vi "GetMoreGitInfoFromHash.vi"(10 "git hash":string, 11 "git hash file path":path=path "C:/Users/jmckenna/MIDAS_GEM_LabVIEW/.git/HEAD/refs/heads/master\n") -> (3 "git commit":T1, 4 "Full git text (before split into cluster)":string)   [LabVIEW 2018]
uses:
  GitCommitData.ctl
  <userlib>/_RADE/MTA-lib/file/file.llb/Valid Path - Traditional__ogtk.vi
  <userlib>/_RADE/MTA-lib/file/file.llb/Strip Path - Traditional__ogtk.vi
panel:
  out "Commit message":string
  out "Date (UTC)":i32
  out "after substring":string
  out "Author email":string
  out "Author name":string
  out "git hash (if matched)":string
  out "Branch":string
  out "stripped path":path
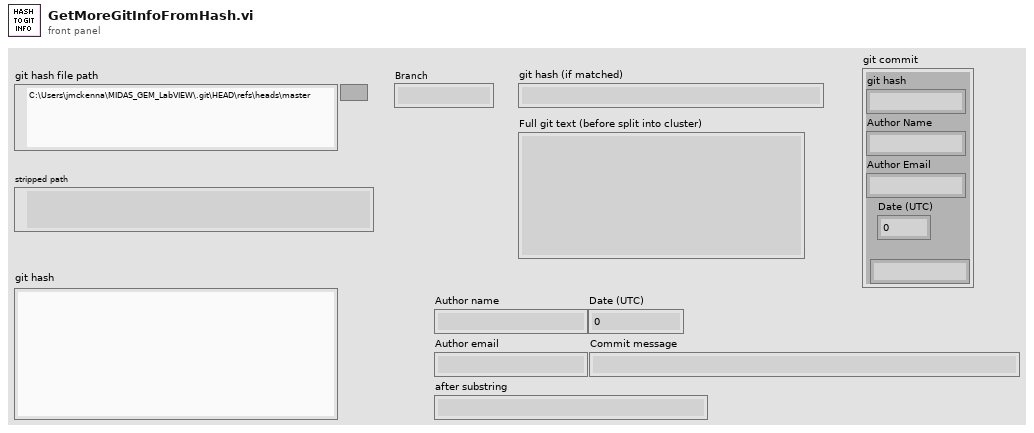
[diagram p1: front panel]
types:
  T1 = typedef "GitCommitData.ctl" = cluster{"git hash":string, "Author Name":string, "Author Email":string, "Date (UTC)":i32, "Commit Message":string}
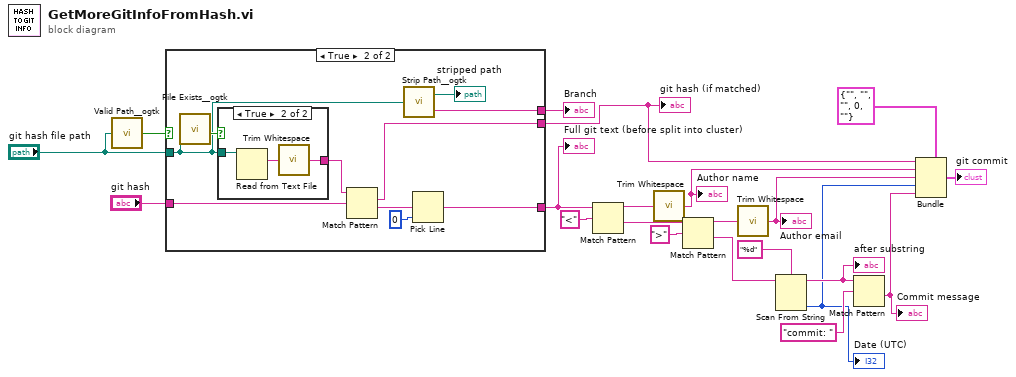
[diagram p0: block diagram]
diagram:
  n1 = call-poly <userlib>:"Valid Path__ogtk.vi"("path"="git hash file path") -> ("valid"=w21:bool)
  n2 = case shown="True" w21 {
    tunnel: "git hash file path" -> [_ w29]
    tunnel: [_ w28] -> w19
    tunnel: "git hash" -> [_ w26]
    tunnel: [_ w24] -> w17
    tunnel: [_ w22] -> w7
    frame False {
    }
    frame True {
      n3 = call <userlib>:"File Exists__ogtk.vi"("file path"=w29) -> ("exists"=w31:bool)  [unwired: 6 in, 1 out]
      n4 = case shown="True" w31 {
        tunnel: w29 -> [_ w34]
        tunnel: [_ w32] -> w27
        frame False {
        }
        frame True {
          n5 = Read from Text File(file (use dialog)=w34) -> (text=w33:string)  [unwired: 3 in, 3 out]
          n6 = call <vilib>:"Trim Whitespace.vi"("string"=w33) -> ("trimmed string"=w32:string)  [unwired: 1 in]
        }
      }
      n7 = Match Pattern(string=w27, regular expression=w26) -> (match substring=w22:string, after substring=w23:string)  [unwired: 1 in, 2 out]
      n8 = call-poly <userlib>:"Strip Path__ogtk.vi"("path"=w29) -> ("stripped path"=→"stripped path":path, "name"=w28:string)
      n9 = Pick Line(multi-line string=w23, line index=0) -> (output string=w24:string)  [unwired: 1 in]
    }
  }
  "Branch" <- w19
  "Full git text (before split into cluster)" <- w17
  "git hash (if matched)" <- w7
  n10 = Match Pattern(string=w17, regular expression="<") -> (before substring=w13:string, after substring=w14:string)  [unwired: 1 in, 2 out]
  n11 = call <vilib>:"Trim Whitespace.vi"("string"=w13) -> ("trimmed string"=w6:string)  [unwired: 1 in]
  "Author name" <- w6
  n12 = Match Pattern(string=w14, regular expression=">") -> (before substring=w12:string, after substring=w11:string)  [unwired: 1 in, 2 out]
  n13 = call <vilib>:"Trim Whitespace.vi"("string"=w12) -> ("trimmed string"=w5:string)  [unwired: 1 in]
  "Author email" <- w5
  n14 = Scan From String(format string="%d", input string=w11) -> (remaining string=w8:string, output 1=w4:i32)  [unwired: 3 in, 2 out]
  "after substring" <- w8
  "Date (UTC)" <- w4
  n15 = Match Pattern(string=w8, regular expression="commit: ") -> (after substring=w3:string)  [unwired: 1 in, 3 out]
  "Commit message" <- w3
  n16 = Bundle(cluster=T1 {"git hash"="", "Author Name"="", "Author Email"="", "Date (UTC)"=0, "Commit Message"=""} ("output cluster"), "git hash"=w7, "Author Name"=w6, "Author Email"=w5, "Date (UTC)"=w4, "Commit Message"=w3) -> (→"git commit":T1)
